vi "MeasLeakRate_v21.vi"() -> ()   [LabVIEW 2011]
uses:
  <vilib>/Analysis/NI_AALPro.lvlib
panel:
  out "Pfit array":dbl[](array[numeric])
  out "tFit array":dbl[](array[numeric])
  in  "tFit":dbl
  out "leak rate":dbl
  out "Polynomial Coefficients":dbl[](array[numeric])
  out "Best Polynomial Fit":dbl[](array[numeric])=[-1.4185856873488687, -1.6139263817489564, -1.4535753275096295, -0.934721257482187, -0.06084472416107456, 1.168009538292087, 2.7539547788012695, 4.6979090060566655, 6.9965349595828625, 9.65378216839643, 12.656869913925354, 16.032582856357365, 19.766321537116767, 23.839791139200322, 28.29201256813708, 33.090057519195085, 38.231169600301214, 43.741895001434145, 49.604230522561835, 55.817258155180305, 63.621549699110574, 70.69684374251437, 78.07805746158404, 85.78401348130417, 93.89514333055536, 102.37353612475415, 111.1585051750553, 120.33168859799997, 129.86351160527155, 139.71949074374146, 149.9584374415381, 160.56464392932688, 171.50086747103902, 182.82343196442633, 194.50463604214053, 206.47125485701025, 218.94296295023602, 231.70008578092185, 244.74755627283324, 258.3136303817438]
  out "weight array":dbl[](array[numeric])
  out "dtArray":dbl[](array[numeric])
  out "t_array":dbl[](array[numeric])
  out "P_array":dbl[](array[numeric])
  in  "# of points to fit":i32=60
  out "angle (°)":dbl
  out "Status":string
  out "error out":errorcluster
  out "T-T0,P":cluster{"element":dbl, "element":dbl}[](array[cluster])
  out "XY Graph":cluster{"Value":dbl[], "Value":dbl[]}[](graph)
  out "T,P":cluster{"element":dbl, "element":dbl}[](array[cluster])
  in  "Control Valve Local":bool
  in  "Exhaust Close":bool
  in  "Exhaust Open":bool
  in  "Control Close":bool
  in  "Control Open":bool
  in  "reset":bool
  in  "# points to watch":i32=60
  out "leak rate (torr/min)":string
  out "P":dbl
  out "first":bool=TRUE
  in  "interval (s)":dbl=0.5
  in  "stop":bool
  out "P(torr)":string
  # "Pressure control valve:"
  # "Exahaust valve:"
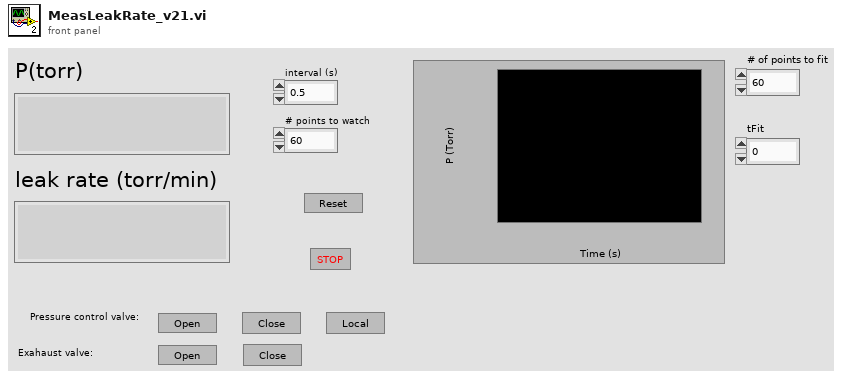
[diagram p1: front panel]
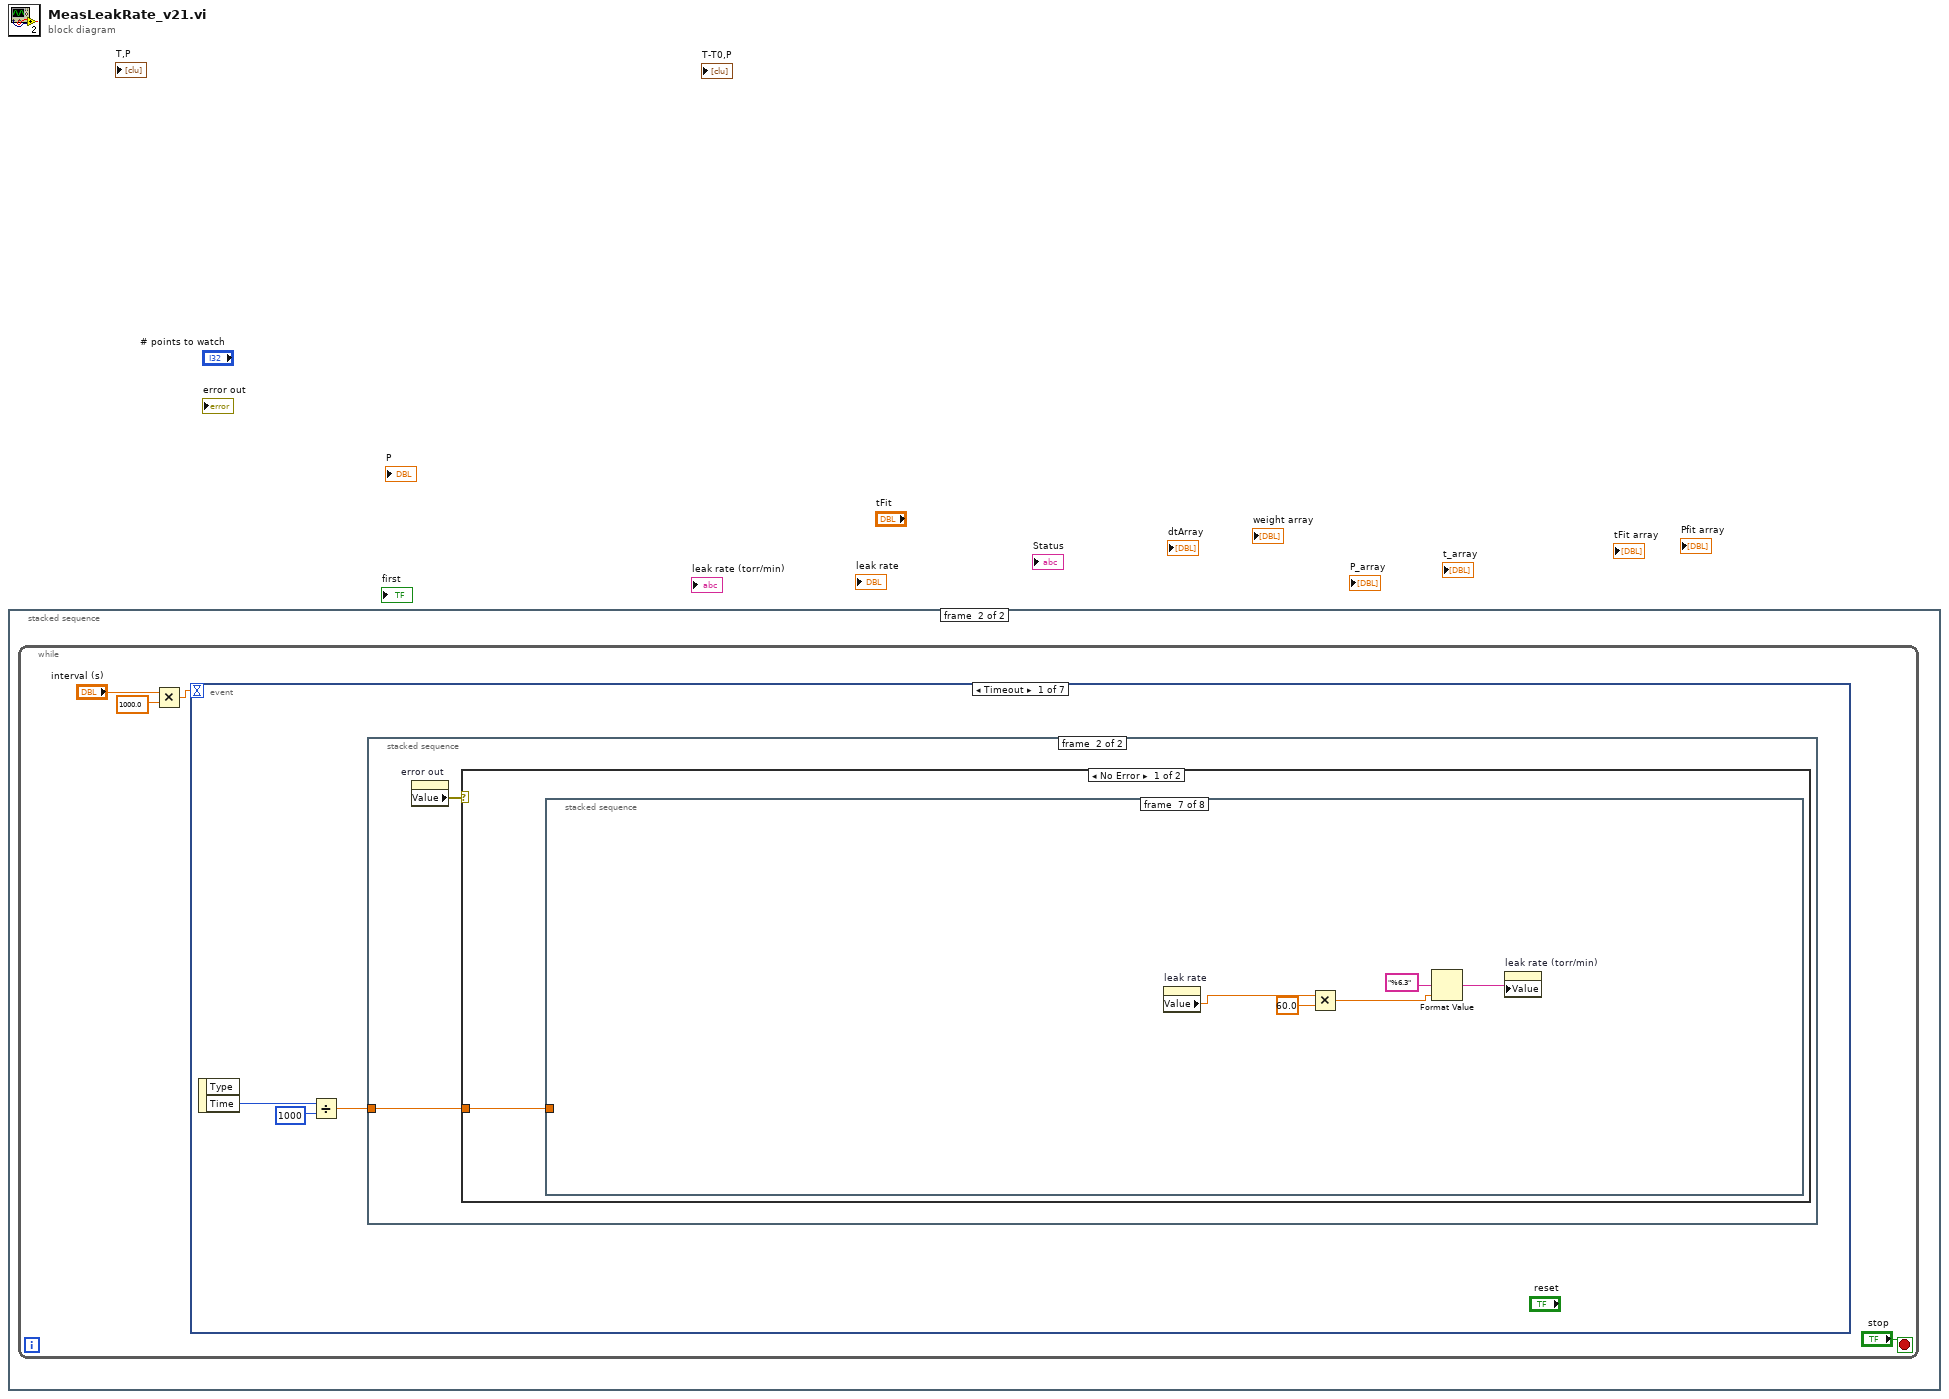
[diagram p0: block diagram]
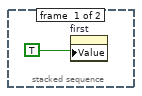
[diagram p2: hidden frame]
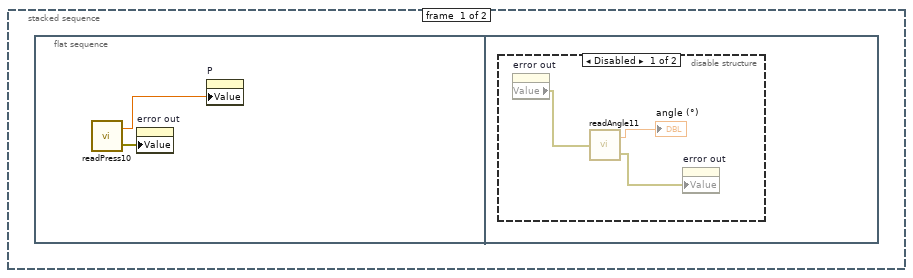
[diagram p3: hidden frame]
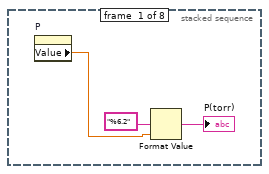
[diagram p5: hidden frame]
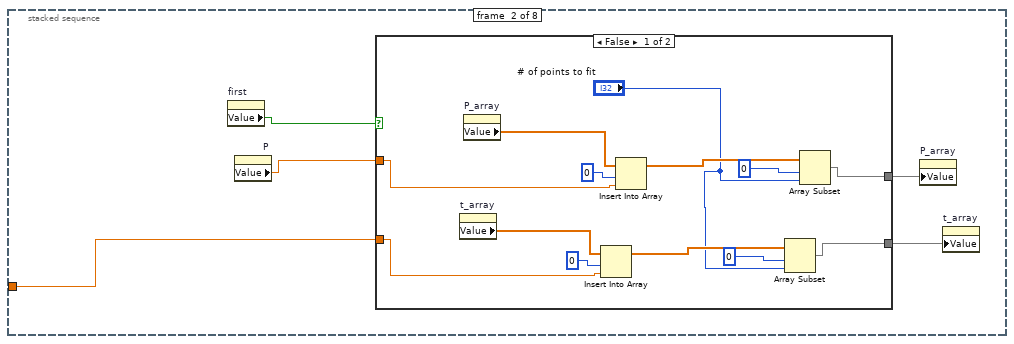
[diagram p6: hidden frame]
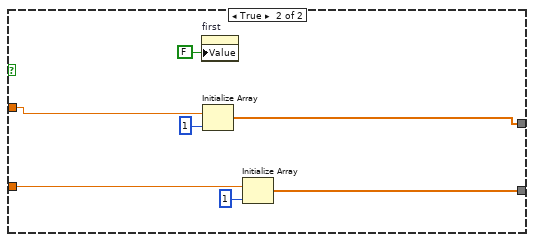
[diagram p7: hidden frame]
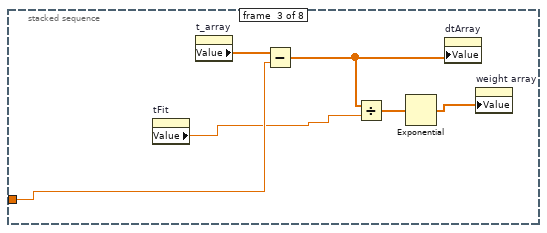
[diagram p8: hidden frame]
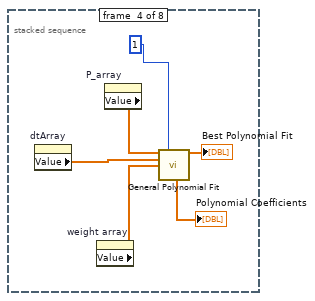
[diagram p9: hidden frame]
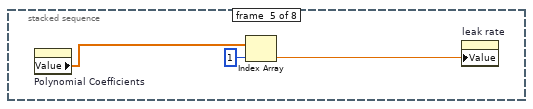
[diagram p10: hidden frame]
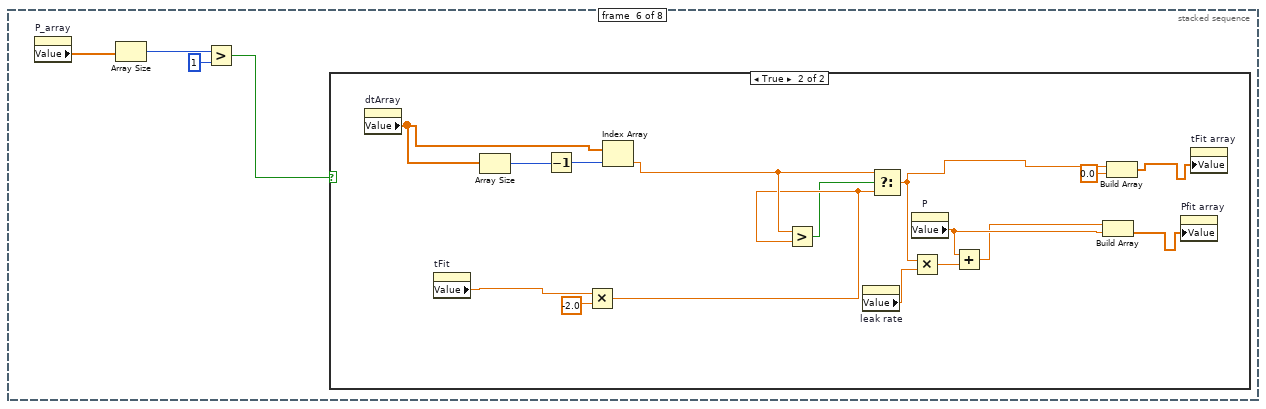
[diagram p11: hidden frame]
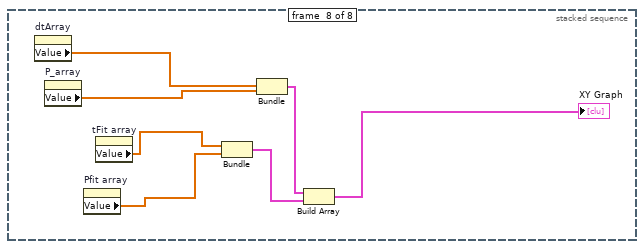
[diagram p13: hidden frame]
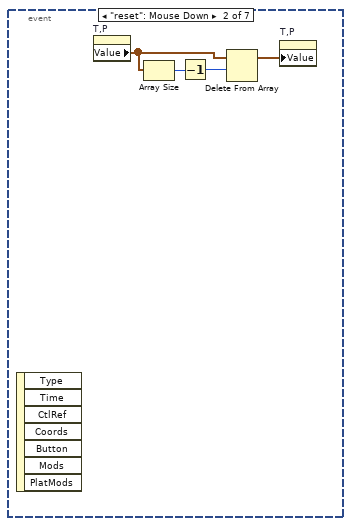
[diagram p15: hidden frame]
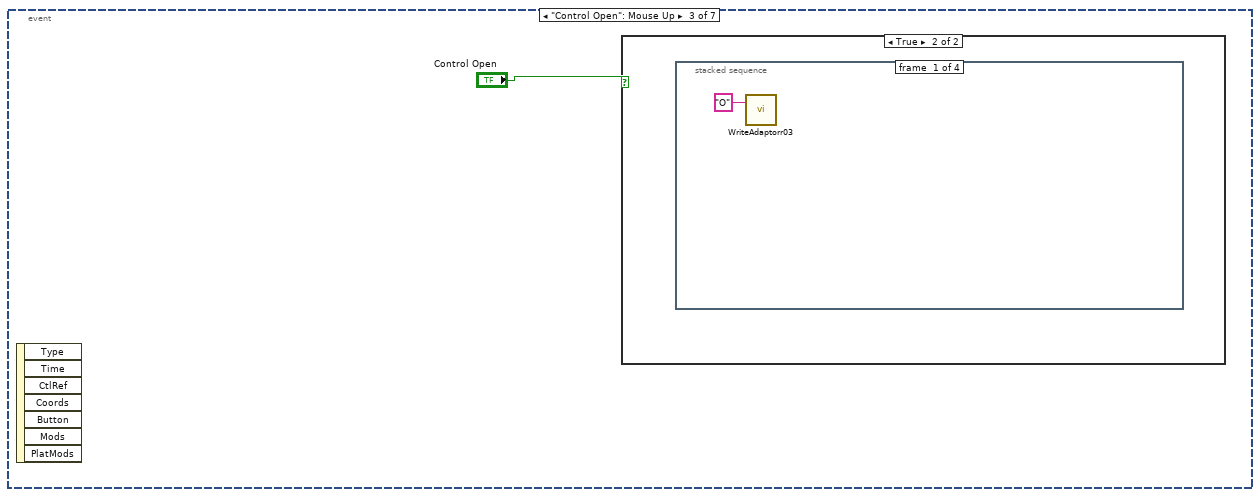
[diagram p16: hidden frame]
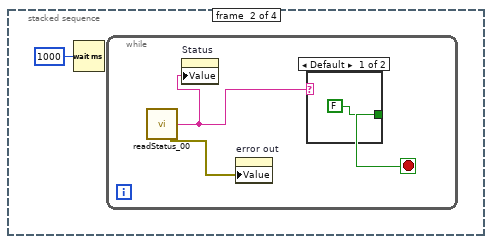
[diagram p18: hidden frame]
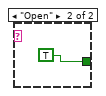
[diagram p19: hidden frame]
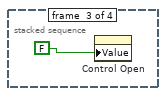
[diagram p20: hidden frame]
diagram:
  n1 = stacked-sequence {
    frame #0 {
      n2 = property on="first" class="Bool (strict)"("Value"=TRUE ("first")) -> ()  [unwired: 2 in, 2 out]
    }
    frame #1 {
      n3 = while {
        stop <- "stop" stop-if-true
        n4 = Multiply(x="interval (s)", y=1000.0) -> (x*y=w3:dbl)
        n5 = event shown="[0] Timeout" {
          selector: _ -> [_ _ _ _ _ _ _]
          dyn-events: _ -> [_ _ _ _ _ _ _]
          timeout: w3 -> [_ _ _ _ _ _ _]
          event Timeout {
            n6 = event-data() -> ("Time"=w8:u32)  [unwired: 1 in, 1 out]
            n7 = Divide(x=w8, y=u32 1000) -> (x/y=w6:dbl)
            n8 = stacked-sequence {
              tunnel: w6 -> [_ w14]
              frame #0 {
                n9 = flat-sequence {
                  frame #0 {
                    n10 = call "readPress10.vi"() -> ("P"=w10:dbl, "error out"=w9:errorcluster)  [unwired: 1 in]
                    n11 = property on="error out" class="Clust (strict)"("Value"=w9) -> ()  [unwired: 2 in, 2 out]
                    n12 = property on="P" class="DigNum (strict)"("Value"=w10) -> ()  [unwired: 2 in, 2 out]
                  }
                  frame #1 {
                    n13 = disable-structure shown="Disabled" {
                      frame Disabled {
                        n14 = property on="error out" class="Clust (strict)"() -> ("Value"=w12:errorcluster)  [unwired: 2 in, 2 out]
                        n15 = call "readAngle11.vi"("error in"=w12) -> ("angle"=→"angle (°)":dbl, "error out"=w11:errorcluster)
                        n16 = property on="error out" class="Clust (strict)"("Value"=w11) -> ()  [unwired: 2 in, 2 out]
                      }
                      frame Enabled {
                      }
                    }
                  }
                }
              }
              frame #1 {
                n17 = property on="error out" class="Clust (strict)"() -> ("Value"=w15:errorcluster)  [unwired: 2 in, 2 out]
                n18 = case shown="No Error" w15 {
                  tunnel: w14 -> [w16 _]
                  frame No Error {
                    n19 = stacked-sequence {
                      tunnel: w16 -> [_ w21 w48 _ _ _ _ _]
                      frame #0 {
                        n20 = property on="P" class="DigNum (strict)"() -> ("Value"=w17:dbl)  [unwired: 2 in, 2 out]
                        n21 = Format Value(format string="%6.2", value (0)=w17) -> (output string=→"P(torr)":string)  [unwired: 1 in]
                      }
                      frame #1 {
                        n22 = property on="first" class="Bool (strict)"() -> ("Value"=w24:bool)  [unwired: 2 in, 2 out]
                        n23 = property on="P" class="DigNum (strict)"() -> ("Value"=w23:dbl)  [unwired: 2 in, 2 out]
                        n24 = case shown="False" w24 {
                          tunnel: w23 -> [w34 w42]
                          tunnel: [w33 w41] -> w22
                          tunnel: w21 -> [w26 w39]
                          tunnel: [w27 w38] -> w20
                          frame False {
                            n25 = property on="t_array" class="Arr (strict)"() -> ("Value"=w25:dbl[])  [unwired: 2 in, 2 out]
                            n26 = property on="P_array" class="Arr (strict)"() -> ("Value"=w32:dbl[])  [unwired: 2 in, 2 out]
                            n27 = Insert Into Array(array=w25, index=0, new element=w26) -> (w30:dbl[])
                            n28 = Insert Into Array(array=w32, index=0, new element=w34) -> (w36:dbl[])
                            n29 = Array Subset(array=w30, index=0, length="# of points to fit") -> (w27:dbl[])
                            n30 = Array Subset(array=w36, index=0, length="# of points to fit") -> (w33:dbl[])
                          }
                          frame True {
                            n31 = property on="first" class="Bool (strict)"("Value"=FALSE ("first")) -> ()  [unwired: 2 in, 2 out]
                            n32 = Initialize Array(w42, 1 ("dimension size")) -> (w41:dbl[])
                            n33 = Initialize Array(w39, 1 ("dimension size")) -> (w38:dbl[])
                          }
                        }
                        n34 = property on="P_array" class="Arr (strict)"("Value"=w22) -> ()  [unwired: 2 in, 2 out]
                        n35 = property on="t_array" class="Arr (strict)"("Value"=w20) -> ()  [unwired: 2 in, 2 out]
                      }
                      frame #2 {
                        n36 = property on="tFit" class="DigNum (strict)"() -> ("Value"=w45:dbl)  [unwired: 2 in, 2 out]
                        n37 = property on="t_array" class="Arr (strict)"() -> ("Value"=w49:dbl[])  [unwired: 2 in, 2 out]
                        n38 = Subtract(x=w49, y=w48) -> (x-y=w47:dbl[])
                        n39 = Divide(x=w47, y=w45) -> (x/y=w50:dbl[])
                        n40 = Exponential(1:w50) -> (0:w46:dbl[])
                        n41 = property on="dtArray" class="Arr (strict)"("Value"=w47) -> ()  [unwired: 2 in, 2 out]
                        n42 = property on="weight array" class="Arr (strict)"("Value"=w46) -> ()  [unwired: 2 in, 2 out]
                      }
                      frame #3 {
                        n43 = property on="dtArray" class="Arr (strict)"() -> ("Value"=w55:dbl[])  [unwired: 2 in, 2 out]
                        n44 = property on="weight array" class="Arr (strict)"() -> ("Value"=w54:dbl[])  [unwired: 2 in, 2 out]
                        n45 = property on="P_array" class="Arr (strict)"() -> ("Value"=w56:dbl[])  [unwired: 2 in, 2 out]
                        n46 = call <vilib>:"General Polynomial Fit.vi"("Y"=w56, "polynomial order"=1, "X"=w55, "Weight"=w54) -> ("Best Polynomial Fit"=→"Best Polynomial Fit":dbl[], "Polynomial Coefficients"=→"Polynomial Coefficients":dbl[])  [unwired: 8 in, 2 out]
                      }
                      frame #4 {
                        n47 = property on="Polynomial Coefficients" class="Arr (strict)"() -> ("Value"=w59:dbl[])  [unwired: 2 in, 2 out]
                        n48 = Index Array(array=w59, index=1) -> (element=w57:dbl)
                        n49 = property on="leak rate" class="DigNum (strict)"("Value"=w57) -> ()  [unwired: 2 in, 2 out]
                      }
                      frame #5 {
                        n50 = property on="P_array" class="Arr (strict)"() -> ("Value"=w60:dbl[])  [unwired: 2 in, 2 out]
                        n51 = Array Size(array=w60) -> (size(s)=w61:i32)
                        n52 = Greater?(x=w61, y=1) -> (0:w63:bool)
                        n53 = case shown="True" w63 {
                          frame False {
                          }
                          frame True {
                            n54 = property on="dtArray" class="Arr (strict)"() -> ("Value"=w73:dbl[])  [unwired: 2 in, 2 out]
                            n55 = property on="tFit" class="DigNum (strict)"() -> ("Value"=w68:dbl)  [unwired: 2 in, 2 out]
                            n56 = Array Size(array=w73) -> (size(s)=w79:i32)
                            n57 = Decrement(x=w79) -> (x-1=w78:i32)
                            n58 = Multiply(x=w68, y=-2.0) -> (x*y=w67:dbl)
                            n59 = Index Array(array=w73, index=w78) -> (element=w74:dbl)
                            n60 = Greater?(x=w74, y=w67) -> (0:w66:bool)
                            n61 = property on="leak rate" class="DigNum (strict)"() -> ("Value"=w77:dbl)  [unwired: 2 in, 2 out]
                            n62 = Select(t=w74, s=w66, f=w67) -> (s? t:f=w70:dbl)
                            n63 = property on="P" class="DigNum (strict)"() -> ("Value"=w72:dbl)  [unwired: 2 in, 2 out]
                            n64 = Multiply(x=w70, y=w77) -> (x*y=w76:dbl)
                            n65 = Add(x=w72, y=w76) -> (x+y=w71:dbl)
                            n66 = Build Array(w71, w72) -> (w64:dbl[])
                            n67 = Build Array(w70, 0.0 ("element")) -> (w65:dbl[])
                            n68 = property on="Pfit array" class="Arr (strict)"("Value"=w64) -> ()  [unwired: 2 in, 2 out]
                            n69 = property on="tFit array" class="Arr (strict)"("Value"=w65) -> ()  [unwired: 2 in, 2 out]
                          }
                        }
                      }
                      frame #6 {
                        n70 = property on="leak rate" class="DigNum (strict)"() -> ("Value"=w82:dbl)  [unwired: 2 in, 2 out]
                        n71 = Multiply(x=w82, y=60.0) -> (x*y=w80:dbl)
                        n72 = Format Value(format string="%6.3", value (0)=w80) -> (output string=w84:string)  [unwired: 1 in]
                        n73 = property on="leak rate (torr/min)" class="Str"("Value"=w84) -> ()  [unwired: 2 in, 2 out]
                      }
                      frame #7 {
                        n74 = property on="dtArray" class="Arr (strict)"() -> ("Value"=w88:dbl[])  [unwired: 2 in, 2 out]
                        n75 = property on="P_array" class="Arr (strict)"() -> ("Value"=w89:dbl[])  [unwired: 2 in, 2 out]
                        n76 = property on="Pfit array" class="Arr (strict)"() -> ("Value"=w86:dbl[])  [unwired: 2 in, 2 out]
                        n77 = property on="tFit array" class="Arr (strict)"() -> ("Value"=w87:dbl[])  [unwired: 2 in, 2 out]
                        n78 = Bundle("Value"=w87, "Value"=w86) -> (w85:cluster{"Value":dbl[], "Value":dbl[]})  [unwired: 1 in]
                        n79 = Bundle("Value"=w88, "Value"=w89) -> (w91:cluster{"Value":dbl[], "Value":dbl[]})  [unwired: 1 in]
                        n80 = Build Array(w91, w85) -> (→"XY Graph":cluster{"Value":dbl[], "Value":dbl[]}[])
                      }
                    }
                  }
                  frame Error {
                  }
                }
              }
            }
          }
          event "reset": Mouse Down {
            n81 = event-data() -> ()  [unwired: 1 in, 7 out]
            n82 = property on="T,P" class="Arr (strict)"() -> ("Value"=w93:cluster{"element":dbl, "element":dbl}[])  [unwired: 2 in, 2 out]
            n83 = Array Size(array=w93) -> (size(s)=w95:i32)
            n84 = Decrement(x=w95) -> (x-1=w94:i32)
            n85 = Delete From Array(array=w93, length=w94) -> (array with subset deleted=w92:cluster{"element":dbl, "element":dbl}[])  [unwired: 1 in, 1 out]
            n86 = property on="T,P" class="Arr (strict)"("Value"=w92) -> ()  [unwired: 2 in, 2 out]
          }
          event "Control Open": Mouse Up {
            n87 = event-data() -> ()  [unwired: 1 in, 7 out]
            n88 = case shown="True" "Control Open" {
              frame False {
              }
              frame True {
                n89 = stacked-sequence {
                  frame #0 {
                    n90 = call "WriteAdaptorr03.vi"("string to write"="O") -> ()  [unwired: 1 in, 1 out]
                  }
                  frame #1 {
                    n91 = Wait (ms)(milliseconds to wait=u32 1000) -> ()  [unwired: 1 out]
                    n92 = while {
                      stop <- w100 stop-if-true
                      n93 = call "readStatus_00.vi"() -> ("Status"=w99:string, "error out"=w101:errorcluster)  [unwired: 1 in, 1 out]
                      n94 = property on="Status" class="Str"("Value"=w99) -> ()  [unwired: 2 in, 2 out]
                      n95 = property on="error out" class="Clust (strict)"("Value"=w101) -> ()  [unwired: 2 in, 2 out]
                      n96 = case shown="Default" w99 {
                        tunnel: [FALSE TRUE] -> w100
                        frame Default {
                        }
                        frame "Open" {
                        }
                      }
                    }
                  }
                  frame #2 {
                    n97 = property on="Control Open" class="Bool (strict)"("Value"=FALSE) -> ()  [unwired: 2 in, 2 out]
                  }
                  frame #3 {
                    n98 = call "WriteAdaptorr03.vi"("string to write"="D5") -> ()  [unwired: 1 in, 1 out]
                  }
                }
              }
            }
          }
          event "Control Close": Mouse Up {
            n99 = event-data() -> ()  [unwired: 1 in, 7 out]
            n100 = case shown="True" "Control Close" {
              frame False {
              }
              frame True {
                n101 = stacked-sequence {
                  frame #0 {
                    n102 = call "WriteAdaptorr03.vi"("string to write"="C") -> ()  [unwired: 1 in, 1 out]
                  }
                  frame #1 {
                    n103 = while {
                      stop <- w110 stop-if-true
                      n104 = call "readStatus_00.vi"() -> ("Status"=w108:string, "error out"=w109:errorcluster)  [unwired: 1 in, 1 out]
                      n105 = property on="Status" class="Str"("Value"=w108) -> ()  [unwired: 2 in, 2 out]
                      n106 = property on="error out" class="Clust (strict)"("Value"=w109) -> ()  [unwired: 2 in, 2 out]
                      n107 = case shown="\"Closed\"" w108 {
                        tunnel: [FALSE TRUE] -> w110
                        frame Default {
                        }
                        frame "Closed" {
                        }
                      }
                    }
                  }
                  frame #2 {
                    n108 = property on="Control Close" class="Bool (strict)"("Value"=FALSE) -> ()  [unwired: 2 in, 2 out]
                  }
                  frame #3 {
                    n109 = call "WriteAdaptorr03.vi"("string to write"="D5") -> ()  [unwired: 1 in, 1 out]
                  }
                }
              }
            }
          }
          event "Exhaust Open": Mouse Up {
            n110 = event-data() -> ()  [unwired: 1 in, 7 out]
            n111 = case shown="True" "Exhaust Open" {
              frame False {
              }
              frame True {
                n112 = call "set_vacuum.vi"("Remote"=TRUE ("Vac Remote"), "Atm"=FALSE ("Atm Exhaust"), "Vac Exhaust"=TRUE) -> ()
              }
            }
          }
          event "Exhaust Close": Mouse Up {
            n113 = event-data() -> ()  [unwired: 1 in, 7 out]
            n114 = case shown="True" "Exhaust Close" {
              frame False {
              }
              frame True {
                n115 = call "set_vacuum.vi"("Remote"=TRUE ("Vac Remote"), "Atm"=FALSE ("Atm Exhaust"), "Vac Exhaust"=FALSE) -> ()
              }
            }
          }
          event "Control Valve Local": Mouse Up {
            n116 = event-data() -> ()  [unwired: 1 in, 7 out]
            n117 = case shown="True" "Control Valve Local" {
              frame False {
              }
              frame True {
                n118 = call "WriteAdaptorr03.vi"("string to write"="D5") -> ()  [unwired: 1 in, 1 out]
              }
            }
          }
        }
      }
    }
  }
